vi "SpinIgualAUmLouco.vi"(11 "Robot in":T1) -> (3 "Cluster de saída":T1)   [LabVIEW 2018]
uses:
  Core/AI Robot.ctl
  Intel/Functions Enum.ctl
  Intel/AttackerStates.ctl
  Path Planning/RRT/PathDests.ctl
  Path Planning/RRT/PathDest.ctl
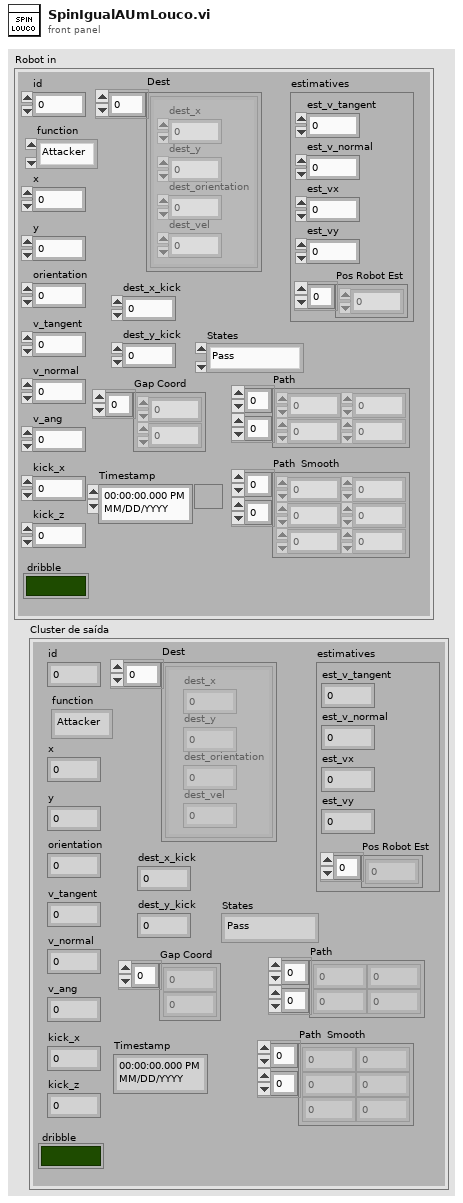
[diagram p1: front panel]
types:
  T1 = typedef "AI Robot.ctl" = cluster{"id":u32, "function":T2, "x":dbl, "y":dbl, "orientation":dbl, "v_tangent":dbl, "v_normal":dbl, "v_ang":dbl, "kick_x":dbl, "kick_z":dbl, "dribble":bool, "Timestamp":timestamp, "estimatives":cluster{"est_v_tangent":dbl, "est_v_normal":dbl, "est_vx":dbl, "est_vy":dbl, "Pos Robot Est":dbl[]}, "dest_x_kick":dbl, "dest_y_kick":dbl, "Gap Coord":dbl[], "States":T3, "Path ":dbl[][], "Path  Smooth":dbl[][], "Dest":T4}
  T2 = typedef "Functions Enum.ctl" = enum16{"Attacker", "Goalie", "Defender", "Striker", "Goto 0", "Dummy", "Kicker", "ZigZag"}
  T3 = typedef "AttackerStates.ctl" = enum16{"Pass", "GoToTangent", "BallGetting", "GoToKick", "Rotate anti-clockwise", "Rotate Clockwise", ""}
  T4 = typedef "PathDests.ctl" = T5[]
  T5 = typedef "PathDest.ctl" = cluster{"dest_x":dbl, "dest_y":dbl, "dest_orientation":dbl, "dest_vel":dbl}
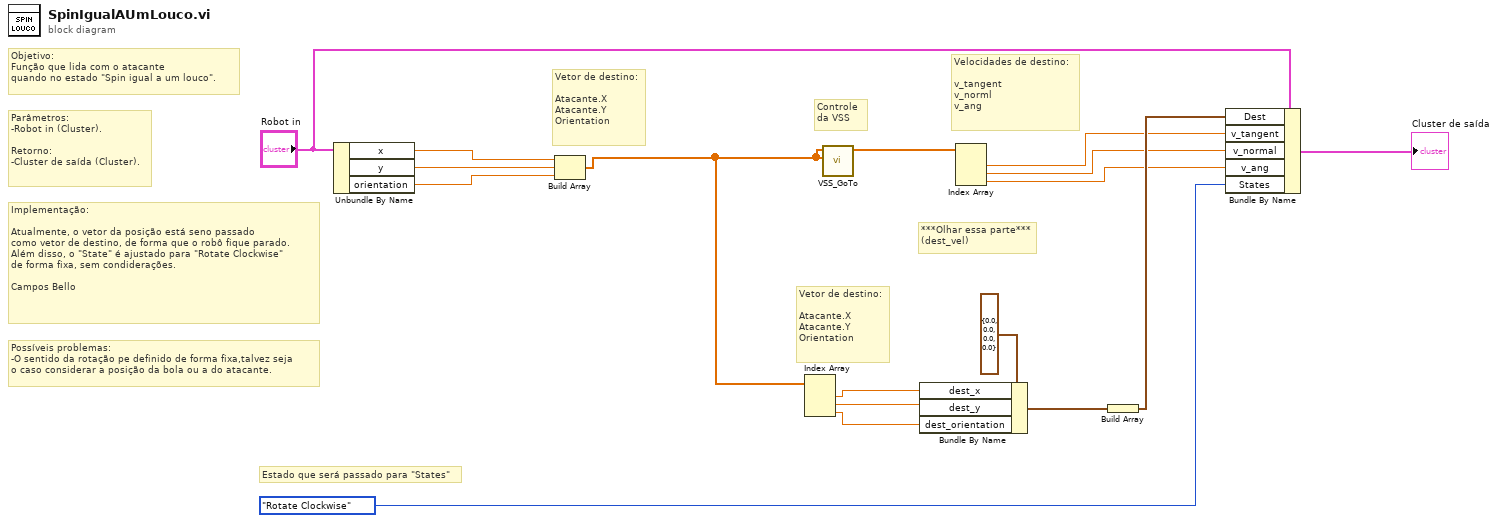
[diagram p0: block diagram]
diagram:
  # "Possíveis problemas:\n-O sentido da rotação pe definido de forma fixa,talvez seja\no caso considerar a posição da bola ou a do atacante."
  # "Implementação:\n\nAtualmente, o vetor da posição está seno passado\ncomo vetor de destino, de forma que o robô fique parado.\nAlém disso, o \"State\" é ajustado para \"Rotate Clockwise\"\nde forma fixa, sem condiderações.\n\nCampos Bello"
  # "Parâmetros:\n-Robot in (Cluster).\n\nRetorno:\n-Cluster de saída (Cluster)."
  # "Objetivo:\nFunção que lida com o atacante\nquando no estado \"Spin igual a um louco\"."
  # "Estado que será passado para \"States\""
  # "Vetor de destino:\n\nAtacante.X\nAtacante.Y\nOrientation"
  # "Velocidades de destino:\n\nv_tangent\nv_norml\nv_ang"
  # "***Olhar essa parte***\n(dest_vel)"
  # "Controle \nda VSS"
  # "Vetor de destino:\n\nAtacante.X\nAtacante.Y\nOrientation"
  n1 = Unbundle By Name("Robot in") -> ("x"=w16:dbl, "y"=w17:dbl, "orientation"=w15:dbl)
  n2 = Build Array(w16, w17, w15) -> (w11:dbl[])
  n3 = Index Array(array=w11) -> (element #1=w10:dbl, element #2=w9:dbl, element #3=w8:dbl)  [unwired: 3 in]
  n4 = call "VSS_GoTo.vi"("SetPoint"=w11, "Position"=w11) -> ("Output Vel"=w12:dbl[])  [unwired: 9 in]
  n5 = Bundle By Name(cluster=T5 {"dest_x"=0.0, "dest_y"=0.0, "dest_orientation"=0.0, "dest_vel"=0.0} ("element"), "dest_x"=w10, "dest_y"=w9, "dest_orientation"=w8) -> (w13:T5)
  n6 = Index Array(array=w12) -> (element #1=w6:dbl, element #2=w5:dbl, element #3=w4:dbl)  [unwired: 3 in]
  n7 = Build Array(w13) -> (w7:T5[])
  n8 = Bundle By Name(cluster="Robot in", "Dest"=w7, "v_tangent"=w6, "v_normal"=w5, "v_ang"=w4, "States"=AttackerStates."Rotate Clockwise") -> (→"Cluster de saída":T1)
